vi "deliver_decision.vi"(9 "deliver":bool, 10 "Position in":T1, 11 "Position":T1) -> (3 "Boolean":bool)   [LabVIEW 2014]
uses:
  <vilib>/Utility/miscctls.llb/LVPositionTypeDef.ctl
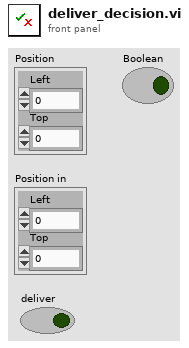
[diagram p1: front panel]
types:
  T1 = typedef "LVPositionTypeDef.ctl" = cluster{"Left":i32, "Top":i32}
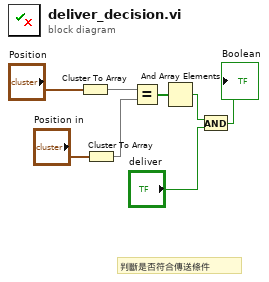
[diagram p0: block diagram]
diagram:
  # "判斷是否符合傳送條件"
  n1 = Cluster To Array(cluster="Position") -> (array=w7:i32[])
  n2 = Cluster To Array(cluster="Position in") -> (array=w8:i32[])
  n3 = Equal?(x=w7, y=w8) -> (x = y?=w2:bool[])
  n4 = And Array Elements(Boolean array=w2) -> (logical AND=w4:bool)
  n5 = And(x=w4, y="deliver") -> (x .and. y?=→"Boolean":bool)
